vi "LSCI332 GetLoopPar.vi"(0 "VISA Rsrc":refnum<visa-resource-name>="GPIB0::12::INSTR", 5 "Boucle(1)":u32(ring) caption="Boucle" items=["Boucle 1", "Boucle 2"], 11 "error in (no error)":errorcluster) -> (4 "Input":u32(ring) caption="Entrée" items=["A", "B", "C", "D"], 6 "Units":u32(ring)=1 caption="Unités du setpoint" items=["Kelvin"=1, "Celsius"=2, "Unités Capteur"=3], 8 "HeatUnits":u32(ring)=1 caption="Unités du chauffage" items=["Courrant"=1, "Puissance"=2], 14 "PowerUp":bool caption="Contrôle actif \nau démarrage", 15 "error out":errorcluster)   [LabVIEW 2019]
doc: "Ce VI lit les paramètres limites de contrôle et ceux de stabilisation du contrôleur."
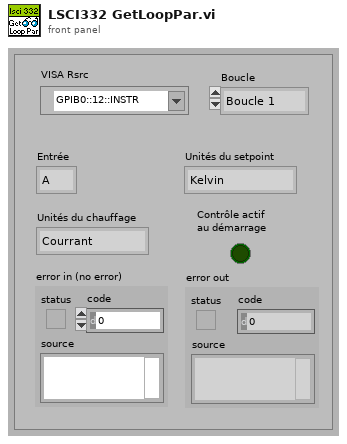
[diagram p1: front panel]
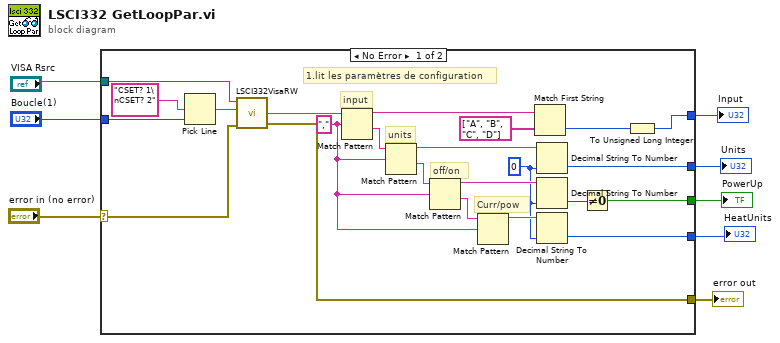
[diagram p0: block diagram]
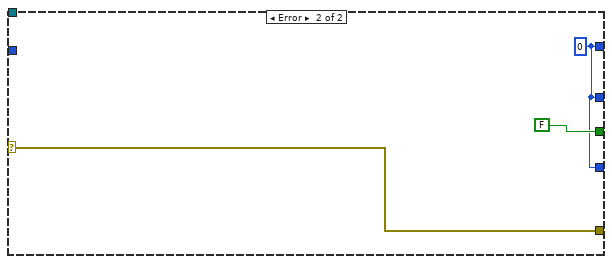
[diagram p2: hidden frame]
diagram:
  n1 = case shown="No Error" "error in (no error)" {
    selector: "error in (no error)" -> [w30 w34]
    tunnel: "VISA Rsrc" -> [w31 _]
    tunnel: "Boucle(1)" -> [w28 _]
    tunnel: [w14 w34] -> w6
    tunnel: [w11 w32] -> w4
    tunnel: [w17 w32] -> w3
    tunnel: [w15 FALSE ("use system decimal point (T)")] -> w2
    tunnel: [w9 w32] -> w1
    frame No Error {
      w18 = u32 0 ("default (0 DBL)")
      w22 = "," ("regular expression")
      # "1.lit les paramètres de configuration"
      # "Curr/pow"
      # "off/on"
      # "units"
      # "input"
      n2 = Pick Line(multi-line string="CSET? 1\nCSET? 2", line index=w28) -> (output string=w27:string)  [unwired: 1 in]
      n3 = call <userlib>:"LSCI332VisaRW.vi"("error in (no error)"=w30, "ChaineCom"=w27, "VISA Rsrc"=w31) -> ("error out"=w14:errorcluster, "ChaineRep"=w26:string)  [unwired: 4 in, 2 out]
      n4 = Match Pattern(string=w26, regular expression=w22) -> (before substring=w12:string, after substring=w24:string)  [unwired: 1 in, 2 out]
      n5 = Match Pattern(string=w24, regular expression=w22) -> (before substring=w19:string, after substring=w25:string)  [unwired: 1 in, 2 out]
      n6 = Match Pattern(string=w25, regular expression=w22) -> (before substring=w20:string, after substring=w23:string)  [unwired: 1 in, 2 out]
      n7 = Match Pattern(string=w23, regular expression=w22) -> (before substring=w21:string)  [unwired: 1 in, 3 out]
      n8 = Match First String(2:string[] ["A", "B", "C", "D"] ("string array"), 3:w12) -> (0:w10:i32)  [unwired: 1 out]
      n9 = Decimal String To Number(string=w19, default (0L)=w18) -> (number=w17:u32)  [unwired: 1 in, 1 out]
      n10 = Decimal String To Number(string=w20, default (0L)=w18) -> (number=w16:u32)  [unwired: 1 in, 1 out]
      n11 = Decimal String To Number(string=w21, default (0L)=w18) -> (number=w9:u32)  [unwired: 1 in, 1 out]
      n12 = Not Equal To 0?(x=w16) -> (x != 0?=w15:bool)
      n13 = To Unsigned Long Integer(number=w10) -> (unsigned 32bit integer=w11:u32)
    }
    frame Error {
      w32 = u32 0
    }
  }
  "error out" <- w6
  "Input" <- w4
  "PowerUp" <- w2
  "Units" <- w3
  "HeatUnits" <- w1
